vi "io_query.vi"(4 "Simulation read buffer (\"Simulation\")":string="Simulation", 5 "Trim Response (F)":bool, 6 "Block Logging (F)":bool, 8 "error in":errorcluster, 9 "Bytes to read (2048)":u32=2048, 10 "write buffer":string, 11 "VISA resource name":refnum<visa-resource-name>) -> (0 "error out":errorcluster, 1 "return count":u32, 2 "read buffer":string, 3 "VISA resource name out":refnum<visa-resource-name>)   [LabVIEW 2014, in "rszvl_rsidr_core.lvlib"]
uses:
  rszvl_rsidr_core.lvlib
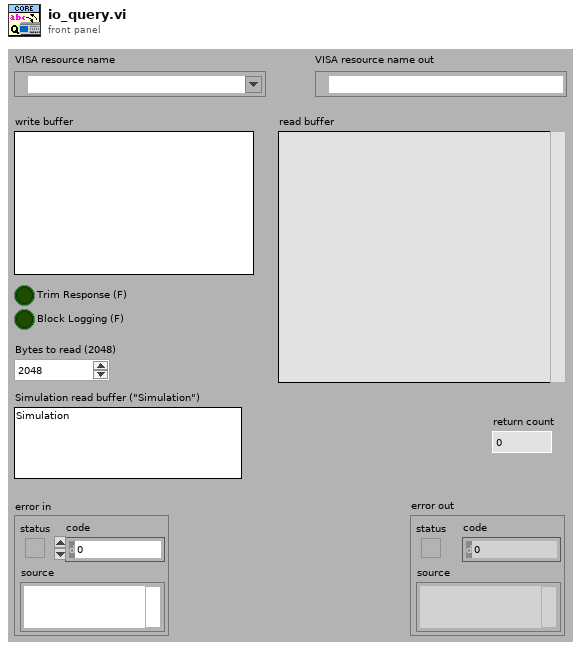
[diagram p1: front panel]
types:
  T1 = typedef "rszvl_rsidr_core.lvlib/type_Session_Data.ctl" = cluster{"Instr type":string, "Instr type for err. msg.":string, "Installed Options":string[], "OPC Timeout":i32, "Query Instrument Status":bool, "Check Range":bool, "Check Options":bool, "Add LF to Write":bool, "Simulate":bool, "Logging":bool, "Logging params":variant, "Interface Type":enum16{"Unknown", "GPIB", "VXI", "GPIB_VXI", "ASRL", "PXI", "TCPIP", "USB", "SOCKET"}, "Fast Sweep":i32, "AdditionalFlags":i32, "WaitBeforeWrite":i32, "WaitBeforeRead":i32, "BinDataChunkSize":i64}
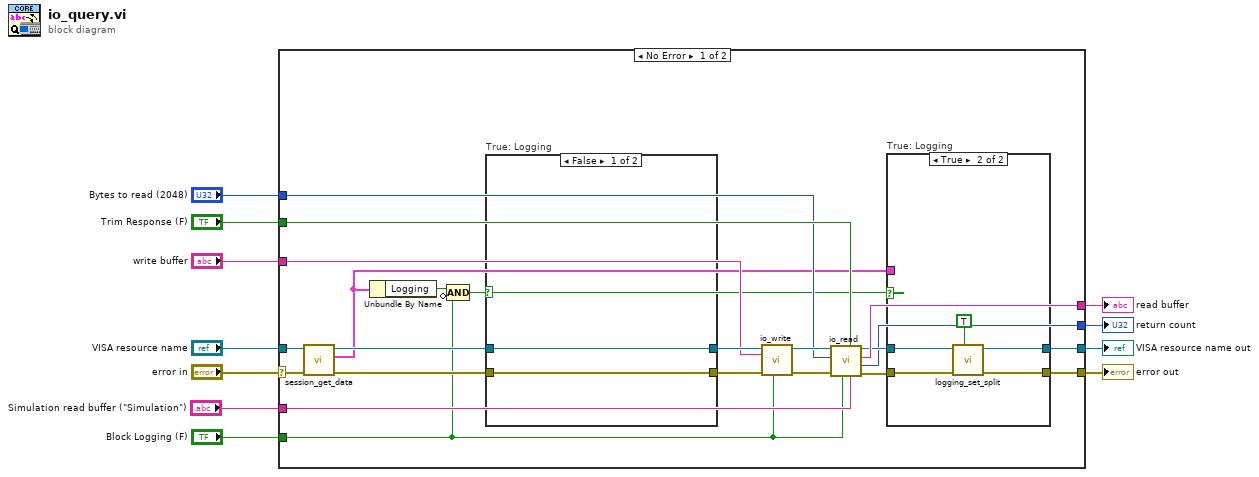
[diagram p0: block diagram]
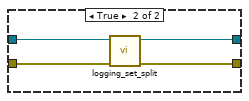
[diagram p3: hidden frame]
diagram:
  n1 = case shown="No Error" "error in" {
    selector: "error in" -> [w25 w48]
    tunnel: [w20 w47] -> w6
    tunnel: [w21 w48] -> w2
    tunnel: "write buffer" -> [w26 _]
    tunnel: "VISA resource name" -> [w24 w47]
    tunnel: "Block Logging (F)" -> [w12 _]
    tunnel: "Bytes to read (2048)" -> [w27 _]
    tunnel: "Simulation read buffer (\"Simulation\")" -> [w16 _]
    tunnel: "Trim Response (F)" -> [w28 _]
    tunnel: [w29 _] -> w5
    tunnel: [w15 _] -> w1
    frame No Error {
      n2 = call "session_get_data.vi"("error in"=w25, "VISA resource name"=w24) -> ("error out"=w23:errorcluster, "Session User Data out"=w17:T1, "VISA resource name out"=w22:refnum<visa-resource-name>)  [unwired: 7 in]
      n3 = Unbundle By Name(w17) -> ("Logging"=w14:bool)
      n4 = Compound Arithmetic op=AND(w14, invert w12) -> (w13:bool)
      n5 = case "True: Logging" shown="False" w13 {
        tunnel: w23 -> [w42 w46]
        tunnel: w22 -> [w41 w45]
        tunnel: [w42 w43] -> w30
        tunnel: [w41 w44] -> w31
        frame False {
        }
        frame True {
          n6 = call "logging_set_split.vi"("error in"=w46, "VISA resource name"=w45) -> ("error out"=w43:errorcluster, "VISA resource name out"=w44:refnum<visa-resource-name>)  [unwired: 8 in]
        }
      }
      n7 = call "io_write.vi"("Block Logging (F)"=w12, "error in"=w30, "write buffer"=w26, "VISA resource name"=w31) -> ("error out"=w32:errorcluster, "VISA resource name out"=w33:refnum<visa-resource-name>)  [unwired: 6 in]
      n8 = call "io_read.vi"("Simulation read buffer (\"Simulation\")"=w16, "Trim Response (F)"=w28, "Block Logging (F)"=w12, "error in"=w32, "byte count (2048)"=w27, "VISA resource name"=w33) -> ("error out"=w19:errorcluster, "return count"=w15:u32, "read buffer"=w29:string, "VISA resource name out"=w18:refnum<visa-resource-name>)  [unwired: 2 in]
      n9 = case "True: Logging" shown="True" w13 {
        tunnel: w19 -> [w35 w40]
        tunnel: [w35 w38] -> w21
        tunnel: w18 -> [w34 w39]
        tunnel: [w34 w37] -> w20
        tunnel: w17 -> [_ _]
        frame False {
        }
        frame True {
          n10 = call "logging_set_split.vi"("Evaluate section error (F)"=TRUE, "error in"=w40, "VISA resource name"=w39) -> ("error out"=w38:errorcluster, "VISA resource name out"=w37:refnum<visa-resource-name>)  [unwired: 7 in]
        }
      }
    }
    frame Error {
    }
  }
  "VISA resource name out" <- w6
  "error out" <- w2
  "read buffer" <- w5
  "return count" <- w1
